vi "ZVL Network Analyser - Init.vi"(8 "error in (no error)":errorcluster) -> (0 "error out":errorcluster, 3 "VISA resource name out":refnum<visa-resource-name>)   [LabVIEW 2019]
uses:
  _Global variables 1.vi
  <instrlib>/rszvl/_utility/rsidr_core.llb/rszvl_rsidr_core.lvlib
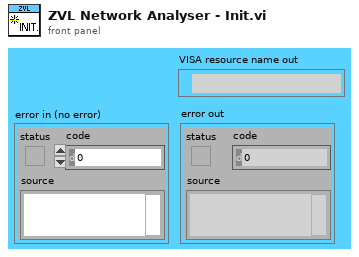
[diagram p1: front panel]
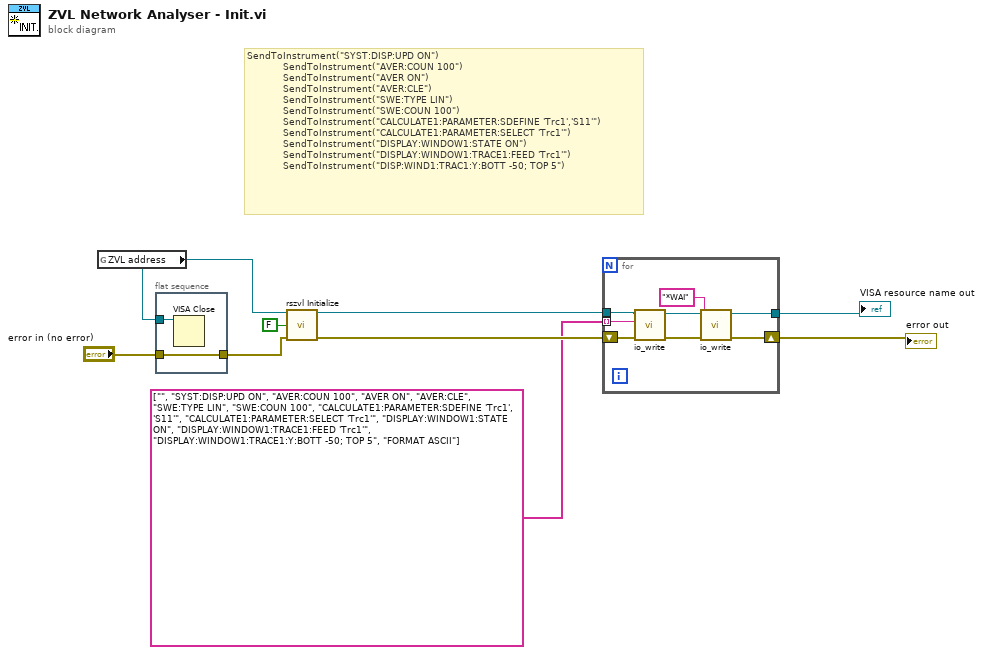
[diagram p0: block diagram]
diagram:
  # "SendToInstrument(\"SYST:DISP:UPD ON\")\n            SendToInstrument(\"AVER:COUN 100\")\n            SendToInstrument(\"AVER ON\")\n            SendToInstrument(\"AVER:CLE\")\n            SendToInstrument(\"SWE:TYPE LIN\")\n            SendToInstrument(\"SWE:COUN 100\")\n            SendToInstrument(\"CALCULATE1:PARAMETER:SDEFINE 'Trc1','S11'\")\n            SendToInstrument(\"CALCULATE1:PARAMETER:SELECT 'Trc1'\")\n            SendToInstrument(\"DISPLAY:WINDOW1:STATE ON\")\n            SendToInstrument(\"DISPLAY:WINDOW1:TRACE1:FEED 'Trc1'\")\n            SendToInstrument(\"DISP:WIND1:TRAC1:Y:BOTT -50; TOP 5\")"
  n1 = global read "_Global variables 1.vi" "ZVL address"() -> (w4:refnum<visa-resource-name>)
  n2 = flat-sequence {
    tunnel: w4 -> [w11]
    tunnel: "error in (no error)" -> [w10]
    tunnel: [w10] -> w2
    frame #0 {
      n3 = VISA Close(VISA resource name=w11) -> ()  [unwired: 1 in, 1 out]
    }
  }
  n4 = call <instrlib>:"rszvl Initialize.vi"("VISA resource name"=w4, "Reset (T: Reset)"=FALSE, "error in (no error)"=w2) -> ("VISA resource name out"=w8:refnum<visa-resource-name>, "error out"=w9:errorcluster)  [unwired: 11 in]
  n5 = for {
    shift-right: [w15] -> w6
    shift-left: w9 -> [w19]
    tunnel: w8 -> [w18]
    tunnel: [w13] -> w7
    tunnel: string[] ["", "SYST:DISP:UPD ON", "AVER:COUN 100", "AVER ON", "AVER:CLE", "SWE:TYPE LIN", "SWE:COUN 100", "CALCULATE1:PARAMETER:SDEFINE 'Trc1', 'S11'", "CALCULATE1:PARAMETER:SELECT 'Trc1'", "DISPLAY:WINDOW1:STATE ON", "DISPLAY:WINDOW1:TRACE1:FEED 'Trc1'", "DISPLAY:WINDOW1:TRACE1:Y:BOTT -50; TOP 5", "FORMAT ASCII"] -> [w17] mode=indexing
    n6 = call <instrlib>:"io_write.vi"("error in"=w19, "write buffer"=w17, "VISA resource name"=w18) -> ("error out"=w16:errorcluster, "VISA resource name out"=w14:refnum<visa-resource-name>)  [unwired: 7 in]
    n7 = call <instrlib>:"io_write.vi"("error in"=w16, "write buffer"="*WAI", "VISA resource name"=w14) -> ("error out"=w15:errorcluster, "VISA resource name out"=w13:refnum<visa-resource-name>)  [unwired: 7 in]
  }
  "VISA resource name out" <- w7
  "error out" <- w6
